vi "deleteGoal.vi"(8 "error in (no error)":errorcluster, 10 "Goal.lvclass":refnum<class "Goal.lvclass">, 11 "Account History in":refnum<class "Account History.lvclass">) -> (0 "error out":errorcluster, 3 "Account History out":refnum<class "Account History.lvclass">)   [LabVIEW 2018, in "Account History.lvclass"]
uses:
  Account History.lvclass
  Goal/Goal.lvclass
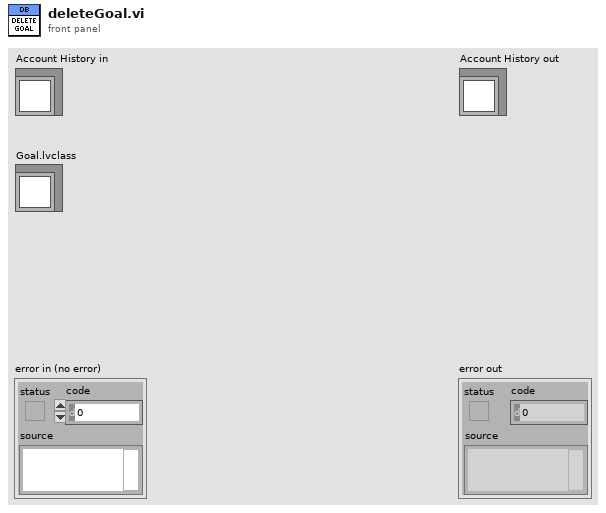
[diagram p1: front panel]
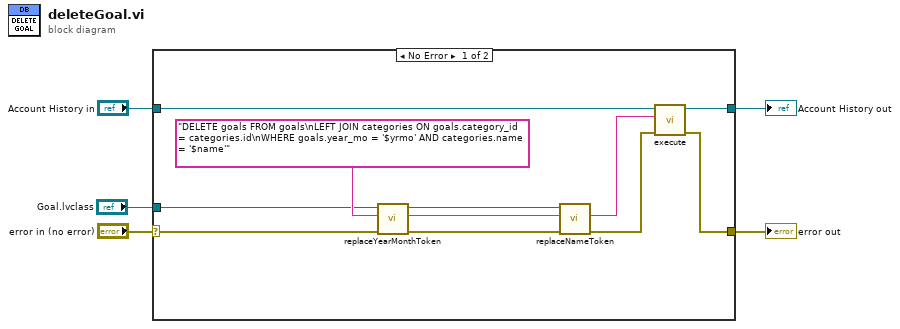
[diagram p0: block diagram]
diagram:
  n1 = case shown="No Error" "error in (no error)" {
    selector: "error in (no error)" -> [w11 w18]
    tunnel: [w14 w18] -> w4
    tunnel: [w15 w17] -> w2
    tunnel: "Account History in" -> [w16 w17]
    tunnel: "Goal.lvclass" -> [w6 _]
    frame No Error {
      n2 = call "replaceYearMonthToken.vi"("error in (no error)"=w11, "Querry In"="DELETE goals FROM goals\nLEFT JOIN categories ON goals.category_id = categories.id\nWHERE goals.year_mo = '$yrmo' AND categories.name = '$name'", "Goal in"=w6) -> ("error out"=w10:errorcluster, "Query Out"=w9:string, "Goal out"=w7:refnum<class "Goal.lvclass">)  [unwired: 6 in]
      n3 = call "replaceNameToken.vi"("error in (no error)"=w10, "Query In"=w9, "Goal in"=w7) -> ("error out"=w12:errorcluster, "Query Out"=w13:string)  [unwired: 6 in, 1 out]
      n4 = call "execute.vi"("error in (no error)"=w12, "SQL query"=w13, "Database in"=w16) -> ("error out"=w14:errorcluster, "Database out"=w15:refnum<class "Account History.lvclass">)  [unwired: 7 in]
    }
    frame Error {
    }
  }
  "error out" <- w4
  "Account History out" <- w2
